vi "LuaVIEW Argument Checking.vi"() -> (0 "pass?":bool)   [LabVIEW 2012]
uses:
  typedefs/t_LuaVIEW Reference.ctl
  subvis/private/LuaVIEW Push (refnum).vi
  subvis/private/LuaVIEW Push (object).vi
panel:
  in  "test script":string="function chk(success)\n  if (success) then error(\"Bad check\") end\nend\n\nnone()\nchk(lv.pcall(none, \"extra\"))\n\nonebool(false)\nonebool(true)\nchk(lv.pcall(onebool,nil))\nchk(lv.pcall(onebool,1))\nchk(lv.pcall(onebool,\"string\"))\nchk(lv.pcall(onebool,obj()))\nchk(lv.pcall(onebool,ref()))\nchk(lv.pcall(onebool,1,1))\n\nonestr(\"string\")\nonestr(1)\nchk(lv.pcall(onestr, \"one\", \"two\"))\nchk(lv.pcall(onestr, obj()))\nchk(lv.pcall(onestr, ref()))\n\nonenum(1)\nonenum(\"1\")\nchk(lv.pcall(onenum, 1, 2))\nchk(lv.pcall(onenum, \"string\"))\nchk(lv.pcall(onenum, true))\nchk(lv.pcall(onenum, ref()))\n\noneobj(obj())\nchk(lv.pcall(oneobj, obj(), obj()))\nchk(lv.pcall(oneobj, 1))\nchk(lv.pcall(oneobj, \"string\"))\nchk(lv.pcall(oneobj, true))\nchk(lv.pcall(oneobj, ref()))\n\noneref(ref())\nchk(lv.pcall(oneref, ref(), ref()))\nchk(lv.pcall(oneref, 1))\nchk(lv.pcall(oneref, \"string\"))\nchk(lv.pcall(oneref, true))\nchk(lv.pcall(oneref, obj()))\n\noneI8(2^7-1)\noneI8(-2^7)\nchk(lv.pcall(oneI8,2^7))\nchk(lv.pcall(oneI8,-2^7-1))\n\noneU8(2^8-1)\noneU8(0)\nchk(lv.pcall(oneU8,2^8))\nchk(lv.pcall(oneU8,-1))\n\noneI16(2^15-1)\noneI16(-2^15)\nchk(lv.pcall(oneI16,2^15))\nchk(lv.pcall(oneI16,-2^15-1))\n\noneU16(2^16-1)\noneU16(0)\nchk(lv.pcall(oneU16,2^16))\nchk(lv.pcall(oneU16,-1))\n\noneI32(2^31-1)\noneI32(-2^31)\nchk(lv.pcall(oneI32,2^31))\nchk(lv.pcall(oneI32,-2^31-1))\n\noneU32(2^32-1)\noneU32(0)\nchk(lv.pcall(oneU32,2^32))\nchk(lv.pcall(oneU32,-1))\n\noneany(nil)\noneany(true)\noneany(1)\noneany(\"string\")\noneany(obj())\noneany(ref())\nchk(lv.pcall(oneany,1,1))\n\nzero_or_one()\nzero_or_one(1)\nchk(lv.pcall(zero_or_one,1,2))\n\nchk(lv.pcall(one_or_two))\none_or_two(1)\none_or_two(1,2)\nchk(lv.pcall(one_or_two,1,2,3))\n\nzero_or_more()\nzero_or_more(1)\nzero_or_more(1,2)\nzero_or_more(1,2,3)\n\nchk(lv.pcall(one_or_more))\none_or_more(1)\none_or_more(1,2)\none_or_more(1,2,3)\n"
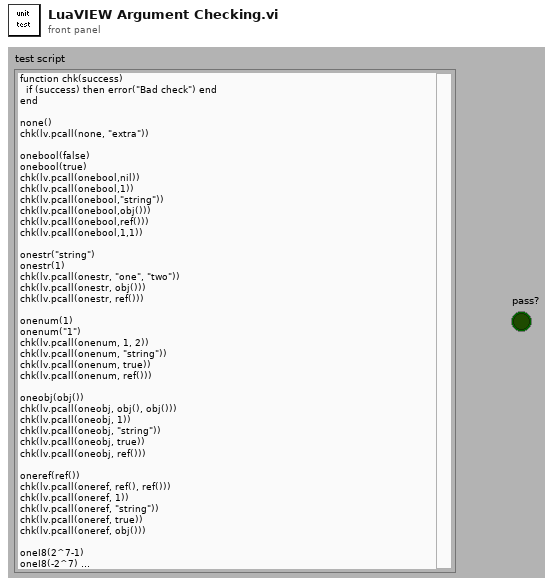
[diagram p1: front panel]
types:
  T1 = enum32{"execute", "initialize", "none()", "onebool(bool:b)", "onestr(str:s)", "onenum(num:n)", "oneobj(obj:o)", "oneref(ref:r)", "oneI8(I8:i)", "oneU8(U8:u)", "oneI16(I16:i)", "oneU16(U16:u)", "oneI32(I32:i)", "oneU32(U32:u)", "oneany(any:a)", "zero_or_one([any:a])", "one_or_two(any:a,[any:a])", "zero_or_more([any:a],...)", "one_or_more(any:a,...)", "obj()", "ref()", "cleanup"}
  T2 = typedef "t_LuaVIEW Reference.ctl" = refnum<k1>
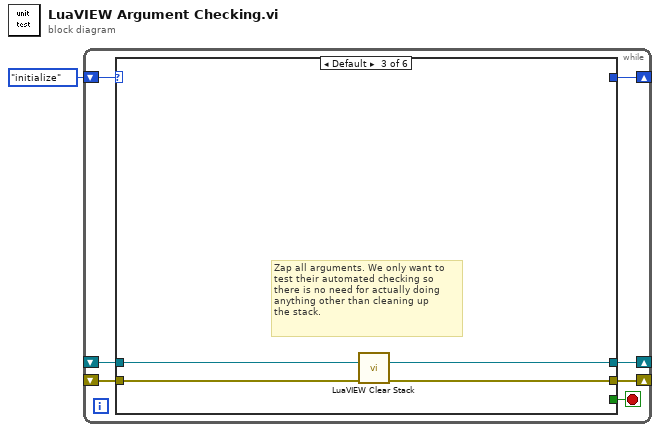
[diagram p0: block diagram]
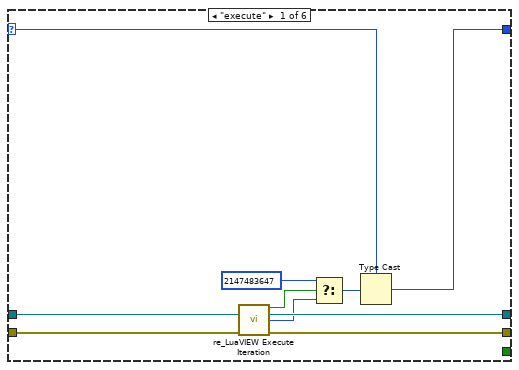
[diagram p2: hidden frame]
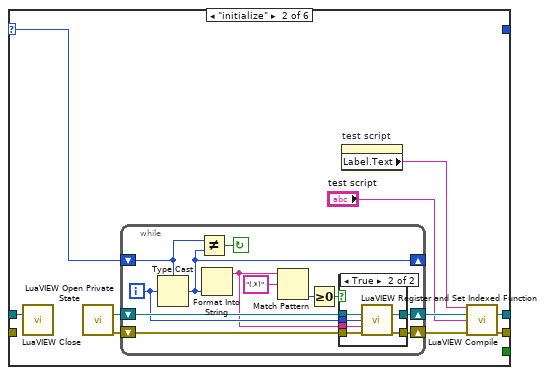
[diagram p3: hidden frame]
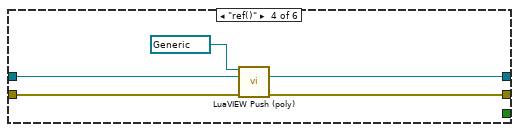
[diagram p5: hidden frame]
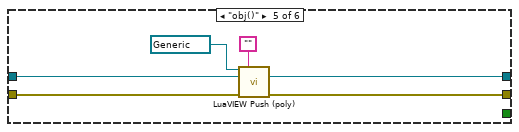
[diagram p6: hidden frame]
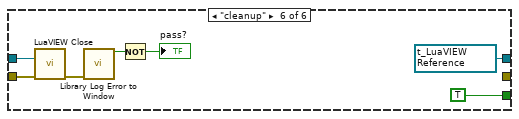
[diagram p7: hidden frame]
diagram:
  n1 = while {
    shift-right: [w6] -> _
    shift-left: T1."initialize" -> [w8]
    shift-right: [w4] -> _
    shift-left: _ -> [w5]
    shift-right: [w3] -> _
    shift-left: _ -> [w2]
    stop <- w7 stop-if-true
    n2 = case shown="Default" w8 {
      selector: w8 -> [w11 w22 _ _ _ _]
      tunnel: [_ _ _ _ _ TRUE] -> w7
      tunnel: [w9 _ _ _ _ _] -> w6
      tunnel: w5 -> [w18 w28 w52 w54 w60 w70]
      tunnel: [w15 w23 w51 w55 w61 w69] -> w4
      tunnel: [w16 w21 w50 w56 w62 _] -> w3
      tunnel: w2 -> [w17 _ w49 w57 w63 w67]
      frame "execute" {
        n3 = call "re_LuaVIEW Execute Iteration.vi"("LuaVIEW reference in"=w18, "init or indexed function error"=w17) -> ("last?"=w13:bool, "LuaVIEW reference out"=w15:T2, "function index"=w14:i32, "final error"=w16:errorcluster)  [unwired: 10 in]
        n4 = Select(t=2147483647, s=w13, f=w14) -> (s? t:f=w10:i32)
        n5 = Type Cast(type=w11, x=w10) -> (*(type *) &x=w9:T1)
      }
      frame "initialize" {
        n6 = call "LuaVIEW Close.vi"("LuaVIEW reference"=w28) -> ()  [unwired: 14 in, 1 out]
        n7 = call "LuaVIEW Open Private State.vi"() -> ("LuaVIEW reference"=w26:T2, "error out"=w27:errorcluster)  [unwired: 14 in]
        n8 = while {
          shift-right: [w34] -> w25
          shift-left: w27 -> [w37]
          shift-right: [w35] -> w24
          shift-left: w26 -> [w36]
          shift-right: [w29] -> _
          shift-left: w22 -> [w30]
          i -> [w33]
          stop <- w40 continue-if-true
          n9 = Type Cast(type=w30, x=w33) -> (*(type *) &x=w29:T1)
          n10 = Not Equal?(x=w30, y=w29) -> (x != y?=w40:bool)
          n11 = Format Into String(w29) -> (resulting string=w31:string)  [unwired: 3 in, 1 out]
          n12 = Match Pattern(string=w31, regular expression="(.*)") -> (offset past match=w38:i32)  [unwired: 1 in, 3 out]
          n13 = Greater Or Equal To 0?(x=w38) -> (x >= 0?=w32:bool)
          n14 = case shown="True" w32 {
            tunnel: w36 -> [w42 w45]
            tunnel: w33 -> [_ w46]
            tunnel: w31 -> [_ w43]
            tunnel: [w41 w48] -> w34
            tunnel: [w42 w47] -> w35
            tunnel: w37 -> [w41 w44]
            frame False {
            }
            frame True {
              n15 = call "LuaVIEW Register and Set Indexed Function.vi"("LuaVIEW reference in"=w45, "index"=w46, "synopsis"=w43, "error in (no error)"=w44) -> ("LuaVIEW reference out"=w47:T2, "error out"=w48:errorcluster)  [unwired: 10 in]
            }
          }
        }
        n16 = property on="test script" class="Str"() -> ("Label.Text"=w19:string)  [unwired: 2 in, 2 out]
        n17 = call "LuaVIEW Compile.vi"("script name"=w19, "LuaVIEW reference in"=w24, "script"="test script", "error in (no error)"=w25) -> ("LuaVIEW reference out"=w23:T2, "error out"=w21:errorcluster)  [unwired: 10 in]
      }
      frame Default {
        # "Zap all arguments. We only want to\ntest their automated checking so\nthere is no need for actually doing\nanything other than cleaning up\nthe stack."
        n18 = call "LuaVIEW Clear Stack.vi"("LuaVIEW reference in"=w52, "error in (no error)"=w49) -> ("LuaVIEW reference out"=w51:T2, "error out"=w50:errorcluster)  [unwired: 12 in]
      }
      frame "ref()" {
        n19 = call-poly "LuaVIEW Push (poly).vi"("refnum"=refnum<vi> refnum, "LuaVIEW reference in"=w54, "error in (no error)"=w57) -> ("LuaVIEW reference out"=w55:T2, "error out"=w56:errorcluster)  [unwired: 11 in]
      }
      frame "obj()" {
        n20 = call-poly "LuaVIEW Push (poly).vi"("object refnum"=refnum<vi> refnum ("refnum"), "method table (use caller's function table)"="", "LuaVIEW reference in"=w60, "error in (no error)"=w63) -> ("LuaVIEW reference out"=w61:T2, "error out"=w62:errorcluster)  [unwired: 10 in]
      }
      frame "cleanup" {
        w69 = T2 refnum items=["LuaVIEW"] ("LuaVIEW reference")
        n21 = call "LuaVIEW Close.vi"("LuaVIEW reference"=w70, "error in (no error)"=w67) -> ("dup error"=w66:errorcluster)  [unwired: 13 in]
        n22 = call "Library Log Error to Window.vi"("error in (no error)"=w66) -> ("error?"=w65:bool)  [unwired: 13 in, 1 out]
        n23 = Not(x=w65) -> (.not. x?=→"pass?":bool)
      }
    }
  }
